vi "SetTrigger.vi"(8 "error in (no error)":errorcluster, 10 "TriggerIn":T1, 11 "CameraSession in":refnum<class "CS250-CameraHardwareClass.lvclass">) -> (0 "error out":errorcluster, 1 "Success":bool, 2 "TriggerOut":T1, 3 "CameraSession out":refnum<class "CS250-CameraHardwareClass.lvclass">)   [LabVIEW 2013, in "CS250-CameraHardwareClass.lvclass"]
uses:
  CS250-CameraHardwareClass.lvclass
  SubVis/TriggerMode_TypDef.ctl
  CS250-CameraHardwareClass.lvclass/CS250-CameraHardwareClass.ctl
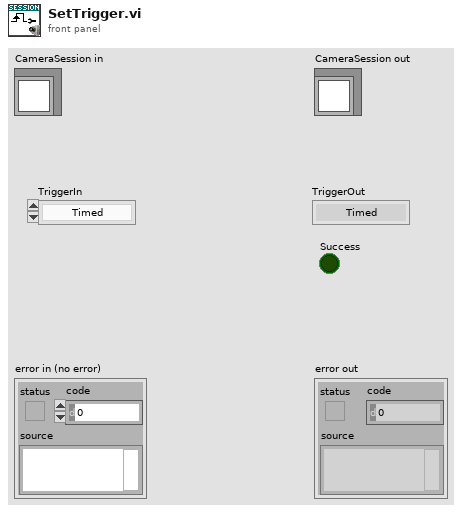
[diagram p1: front panel]
types:
  T1 = typedef "TriggerMode_TypDef.ctl" = enum16{"Timed", "Strobed", "Bulb", "Trigger first", "Flash", "Variable Timed"}
  T2 = typedef "CamCluster.ctl" = cluster{"hcam out":i16, "TempImage":T3, "Pointer":u32, "exp_bytes out":u32, "rgn_array":cluster{"s1":u16, "s2":u16, "sbin":u16, "p1":u16, "p2":u16, "pbin":u16}, "CameraName":string}
  T3 = typedef "IMAQ Image.ctl" = refnum<image>
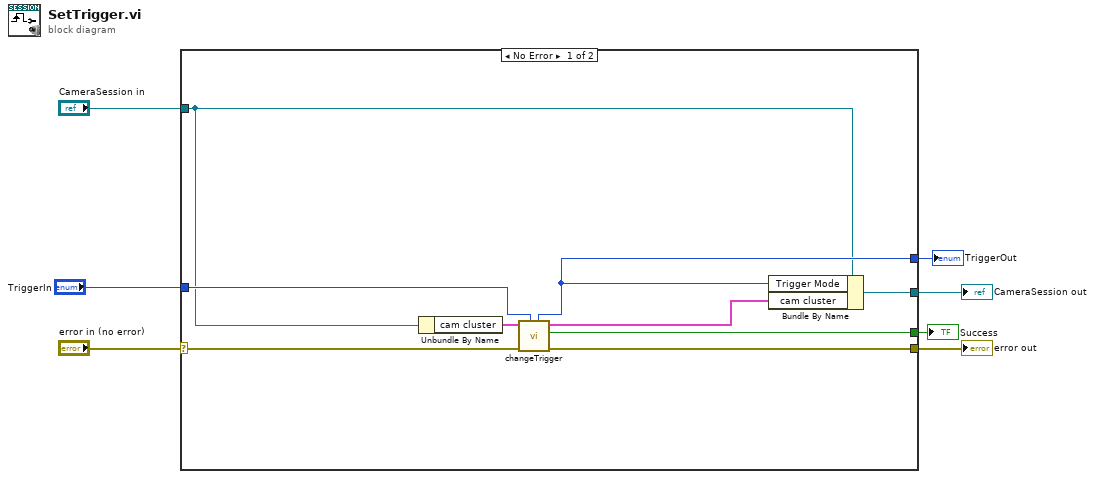
[diagram p0: block diagram]
diagram:
  n1 = case shown="No Error" "error in (no error)" {
    selector: "error in (no error)" -> [w13 w18]
    tunnel: [w12 w18] -> w6
    tunnel: [w15 w17] -> w4
    tunnel: "CameraSession in" -> [w8 w17]
    tunnel: [w11 _] -> w3
    tunnel: [w10 _] -> w2
    tunnel: "TriggerIn" -> [w9 _]
    frame No Error {
      n2 = Unbundle By Name(w8) -> ("cam cluster"=w16:T2)
      n3 = call "changeTrigger.vi"("trigger mode"=w9, "error in (no error)"=w13, "cam cluster out in"=w16) -> ("error out"=w12:errorcluster, "Success"=w11:bool, "cam cluster out"=w14:T2, "trigger mode out"=w10:T1)  [unwired: 5 in]
      n4 = Bundle By Name(cluster=w8, "Trigger Mode"=w10, "cam cluster"=w14) -> (w15:refnum<class "CS250-CameraHardwareClass.lvclass">)
    }
    frame Error {
    }
  }
  "error out" <- w6
  "CameraSession out" <- w4
  "Success" <- w3
  "TriggerOut" <- w2
